vi "LoadConductusLTC-20c.vi"() -> ()   [LabVIEW 2020]
uses:
  <vilib>/Utility/file.llb/Read From Spreadsheet File (DBL).vi
panel:
  in  "Case Constant\n(See Context Help)":bool=TRUE
  out "ManyCal?":string="Too Many Calibration Entries"
  out "Sensor":string=":cernox 1030 X04981.cal2"
  out "Loading:":i32
  in  "More...":bool=TRUE
  out "CalArray":string[](array[string])=["325.000,2.02480,", "320.000,2.02830,", "310.000,2.03560,", "300.000,2.04330,", "290.000,2.05150,", "280.000,2.05960,", "270.000,2.06840,", "260.000,2.07700,", "250.000,2.08660,", "240.000,2.09600,", "230.000,2.10620,", "220.000,2.11640,", "210.000,2.12740,", "200.000,2.13890,", "190.000,2.15060,", "180.000,2.16290,", "170.000,2.17600,", "160.000,2.18960,", "150.000,2.20390,", "140.000,2.21930,", "130.000,2.23510,", "120.000,2.25180,", "110.000,2.26960,", "100.000,2.28870,", "90.000,2.30910,", "80.000,2.33160,", "77.350,2.33790,", "75.000,2.34350,", "70.000,2.35620,", "60.000,2.38390,", "56.000,2.39580,", "54.000,2.40200,", "50.000,2.41500,", "46.000,2.42910,", "44.000,2.43630,", "40.000,2.45170,", "38.000,2.45980,", "36.000,2.46820,", "34.000,2.47700,", "32.000,2.48650,", "30.000,2.49610,", "28.000,2.50610,", "26.000,2.51680,", "24.000,2.52810,", "22.000,2.54030,", "20.000,2.55340,", "19.000,2.56040,", "18.000,2.56750,", "17.000,2.57510,", "16.000,2.58310,", "15.000,2.59170,", "14.000,2.60120,", "13.000,2.61050,", "12.000,2.62100,", "11.000,2.63250,", "10.000,2.64480,", "9.500,2.65150,", "9.000,2.65880,", "8.500,2.66660,", "8.000,2.67440,", "7.500,2.68330,", "7.000,2.69270,", "6.500,2.70230,", "6.000,2.71370,", "5.800,2.71840,", "5.400,2.72870,", "5.000,2.73950,", "4.600,2.75160,", "4.200,2.76480,", "4.000,2.77230,", "3.900,2.77610,", "3.800,2.78000,", "3.700,2.78390,", "3.600,2.78810,", "3.500,2.79240,", "3.400,2.79700,", "3.300,2.80160,", "3.200,2.80650,", "3.100,2.81150,", "3.000,2.81660,", "2.900,2.82200,", "2.800,2.82780,", "2.700,2.83370,", "2.600,2.84000,", "2.500,2.84660,", "2.400,2.85350,", "2.300,2.86120,", "2.200,2.86870,", "2.100,2.87700,", "2.000,2.88560,", "1.900,2.89500,", "1.800,2.90520,", "1.700,2.91630,", "1.600,2.92920,", "1.500,2.94380,", "1.400,2.96020,", "1.300,2.97870,"]
  out "CharMatch":string="SCALT4,2,0,OptCernoxX02158,-1.0,"
  out "TempData":sgl[](array[numeric])=[325.0, 320.0, 310.0, 300.0, 290.0, 280.0, 270.0, 260.0, 250.0, 240.0, 230.0, 220.0, 210.0, 200.0, 190.0, 180.0, 170.0, 160.0, 150.0, 140.0, 130.0, 120.0, 110.0, 100.0, 90.0, 80.0, 77.35, 75.0, 70.0, 60.0, 56.0, 54.0, 50.0, 46.0, 44.0, 40.0, 38.0, 36.0, 34.0, 32.0, 30.0, 28.0, 26.0, 24.0, 22.0, 20.0, 19.0, 18.0, 17.0, 16.0, 15.0, 14.0, 13.0, 12.0, 11.0, 10.0, 9.5, 9.0, 8.5, 8.0, 7.5, 7.0, 6.5, 6.0, 5.8, 5.4, 5.0, 4.6, 4.2, 4.0, 3.9, 3.8, 3.7, 3.6, 3.5, 3.4, 3.3, 3.2, 3.1, 3.0, 2.9, 2.8, 2.7, 2.6, 2.5, 2.4, 2.3, 2.2, 2.1, 2.0, 1.9, 1.8, 1.7, 1.6, 1.5, 1.4, 1.3] format="%.2f"
  out "LogOhms":sgl[](array[numeric])=[2.0248, 2.0283, 2.0356, 2.0433, 2.0515, 2.0596, 2.0684, 2.077, 2.0866, 2.096, 2.1062, 2.1164, 2.1274, 2.1389, 2.1506, 2.1629, 2.176, 2.1896, 2.2039, 2.2193, 2.2351, 2.2518, 2.2696, 2.2887, 2.3091, 2.3316, 2.3379, 2.3435, 2.3562, 2.3839, 2.3958, 2.402, 2.415, 2.4291, 2.4363, 2.4517, 2.4598, 2.4682, 2.477, 2.4865, 2.4961, 2.5061, 2.5168, 2.5281, 2.5403, 2.5534, 2.5604, 2.5675, 2.5751, 2.5831, 2.5917, 2.6012, 2.6105, 2.621, 2.6325, 2.6448, 2.6515, 2.6588, 2.6666, 2.6744, 2.6833, 2.6927, 2.7023, 2.7137, 2.7184, 2.7287, 2.7395, 2.7516, 2.7648, 2.7723, 2.7761, 2.78, 2.7839, 2.7881, 2.7924, 2.797, 2.8016, 2.8065, 2.8115, 2.8166, 2.822, 2.8278, 2.8337, 2.84, 2.8466, 2.8535, 2.8612, 2.8687, 2.877, 2.8856, 2.895, 2.9052, 2.9163, 2.9292, 2.9438, 2.9602, 2.9787] format="%.2f"
  in  "Sensor BasePath":path=path "/Opticsmac/Thermometer Calibrations/ Optics"
  out "Sensor Path":path=path "/Opticsmac/Thermometer Calibrations/ Optics"
  in  "Load Curve":bool
  in  "Sensor Selection":u16(ring) items=["MultiSample30T", "MultiSample20T/Single Sample30T (head..)", "TransmissionProbe 30T", "Double Sample 30T", "SingleSample 30T", "Voigt-6SampleProbe 20T", "Nurmikko30T Top-emission", "Wim MOKE Probe"]
  in  "Sensor Array":T1(array[cluster])=[{"Sensor Path"=path "cernox 1030 X04981.cal2", "Sensor Info"="MultiSample30T"}, {"Sensor Path"=path "NML Opt Cernox X01971.cal", "Sensor Info"="MultiSample20T/Single Sample30T (head..)"}, {"Sensor Path"=path "cernox 1030 (x02158).rev", "Sensor Info"="TransmissionProbe 30T"}, {"Sensor Path"=path "NML-Opt Cernox X02363.cal2", "Sensor Info"="Double Sample 30T"}, {"Sensor Path"=path "", "Sensor Info"="SingleSample 30T"}, {"Sensor Path"=path "", "Sensor Info"="Voigt-6SampleProbe 20T"}, {"Sensor Path"=path "NML-Opt Cernox X04975.cal", "Sensor Info"="Nurmikko30T Top-emission"}, {"Sensor Path"=path "cernox 1010(x01974).rev", "Sensor Info"="Wim MOKE Probe"}]
  in  "LTC-20 BPIB":refnum<visa-resource-name>
  # "Tested successfully on S/N 0195"
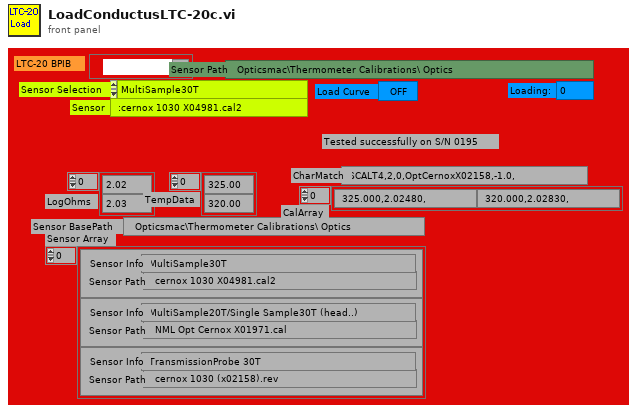
[diagram p1: front panel]
types:
  T1 = cluster{"Sensor Path":path, "Sensor Info":string}[]
  T2 = cluster{"Sensor Path":path, "Sensor Info":string}
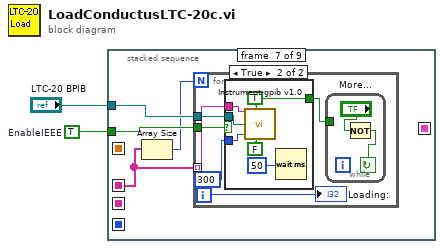
[diagram p0: block diagram]
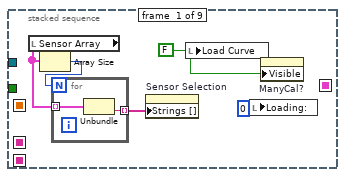
[diagram p2: hidden frame]
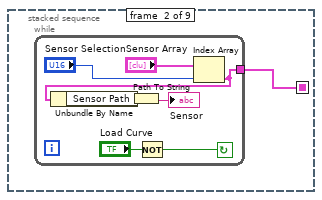
[diagram p3: hidden frame]
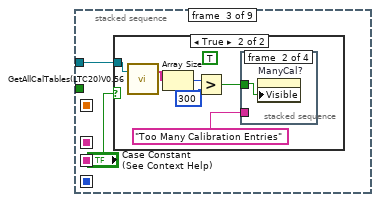
[diagram p4: hidden frame]
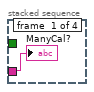
[diagram p6: hidden frame]
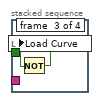
[diagram p7: hidden frame]
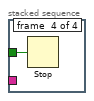
[diagram p8: hidden frame]
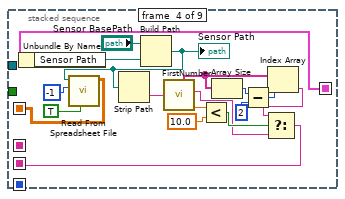
[diagram p9: hidden frame]
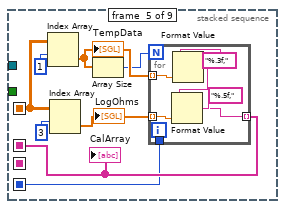
[diagram p10: hidden frame]
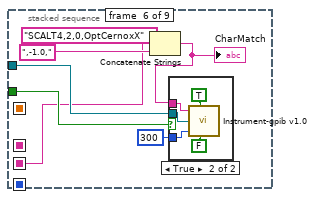
[diagram p11: hidden frame]
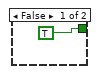
[diagram p13: hidden frame]
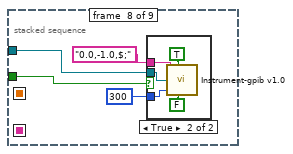
[diagram p14: hidden frame]
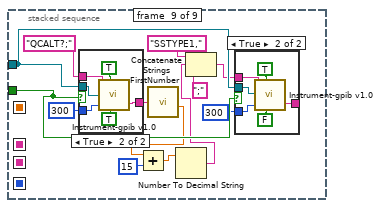
[diagram p16: hidden frame]
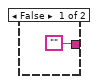
[diagram p17: hidden frame]
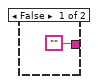
[diagram p18: hidden frame]
diagram:
  w2 = TRUE  # EnableIEEE
  n1 = stacked-sequence {
    seq-local: [_ w10 _ _ _ _ _ _ _] -> [_ _ _ w48 _ _ _ _ _]
    seq-local: [_ _ _ w45 _ _ _ _ _] -> [_ _ _ _ w54 _ _ _ _]
    seq-local: [_ _ _ _ w50 _ _ _ _] -> [_ _ _ _ _ _ w77 _ _]
    seq-local: [_ _ _ w31 _ _ _ _ _] -> [_ _ _ _ _ w65 _ _ _]
    seq-local: [_ _ _ _ w49 _ _ _ _] -> [_ _ _ _ _ _ _ _ _]
    tunnel: w2 -> [_ _ _ _ _ w68 w79 w97 w113]
    tunnel: "LTC-20 BPIB" -> [_ _ w19 _ _ w70 w78 w96 w114]
    frame #0 {
      w4 = FALSE
      n2 = local read "Sensor Array"() -> (w7:T1)
      n3 = Array Size(array=w7) -> (size(s)=w6:i32)
      n4 = for {
        N: w6 -> [_]
        tunnel: w7 -> [w9] mode=indexing
        tunnel: [w8] -> w5 mode=indexing
        n5 = Unbundle(w9) -> ("Sensor Info"=w8:string)  [unwired: 1 out]
      }
      n6 = property on="Sensor Selection" class="Ring (strict)"("Strings []"=w5) -> ()  [unwired: 2 in, 2 out]
      n7 = local write "Load Curve"(w4) -> ()
      n8 = local write "Loading:"(0) -> ()
      n9 = property on="ManyCal?" class="Str"("Visible"=w4) -> ()  [unwired: 2 in, 2 out]
    }
    frame #1 {
      n10 = while {
        tunnel: [w13] -> w10
        stop <- w16 continue-if-true
        n11 = Not(x="Load Curve") -> (.not. x?=w16:bool)
        n12 = Index Array(array="Sensor Array", index="Sensor Selection") -> (element=w13:T2)
        n13 = Unbundle By Name(w13) -> ("Sensor Path"=w12:path)
        n14 = Path To String(path=w12) -> (string=→"Sensor":string)
      }
    }
    frame #2 {
      n15 = case shown="True" "Case Constant\n(See Context Help)" {
        tunnel: w19 -> [_ w24]
        frame False {
        }
        frame True {
          (unwired) TRUE
          n16 = call "GetAllCalTables(LTC20)V0.56.vi"("LTC-20 IEEE"=w24) -> ("CalTables"=w25:string[])  [unwired: 1 in, 1 out]
          n17 = Array Size(array=w25) -> (size(s)=w21:i32)
          n18 = Greater?(x=w21, y=300) -> (0:w20:bool)
          n19 = stacked-sequence {
            tunnel: w20 -> [_ w27 w29 w30]
            tunnel: "Too Many Calibration Entries" -> [w26 _ _ _]
            frame #0 {
              "ManyCal?" <- w26
            }
            frame #1 {
              n20 = property on="ManyCal?" class="Str"("Visible"=w27) -> ()  [unwired: 2 in, 2 out]
            }
            frame #2 {
              n21 = Not(x=w29) -> (.not. x?=w28:bool)
              n22 = local write "Load Curve"(w28) -> ()
            }
            frame #3 {
              n23 = Stop(stop? (T)=w30) -> ()
            }
          }
        }
      }
    }
    frame #3 {
      n24 = Unbundle By Name(w48) -> ("Sensor Path"=w46:path)
      n25 = Build Path(base path="Sensor BasePath", name or relative path=w46) -> (appended path=w42:path)
      "Sensor Path" <- w42
      n26 = call-poly <vilib>:"Read From Spreadsheet File.vi"("transpose (no:F)"=TRUE, "number of rows (all:-1)"=-1, "file path (dialog if empty)"=w42) -> ("all rows"=w45:dbl[][])  [unwired: 4 in, 4 out]
      n27 = Strip Path(path=w42) -> (name=w41:string)  [unwired: 1 out]
      n28 = call "FirstNumber.vi"("Input String"=w41) -> ("Number Stings"=w38:string[], 4:"LastNumber"=w32:string, 6:"LastNumber"=w40:ext)  [unwired: 3 out]
      n29 = Less?(x=w40, y=10.0) -> (x < y?=w34:bool)
      n30 = Array Size(array=w38) -> (size(s)=w36:i32)
      n31 = Subtract(x=w36, y=2) -> (x-y=w37:i32)
      n32 = Index Array(array=w38, index=w37) -> (element=w33:string)
      n33 = Select(t=w33, s=w34, f=w32) -> (s? t:f=w31:string)
    }
    frame #4 {
      n34 = Index Array(array=w54, index (row)=1) -> (element=w53:dbl[])  [unwired: 1 in]
      "TempData" <- w53
      n35 = Index Array(array=w54, index (row)=3) -> (element=w52:dbl[])  [unwired: 1 in]
      "LogOhms" <- w52
      n36 = Array Size(array=w53) -> (size(s)=w51:i32)
      n37 = for {
        N: w51 -> [_]
        tunnel: w53 -> [w58] mode=indexing
        tunnel: w52 -> [w63] mode=indexing
        tunnel: [w60] -> w50 mode=indexing
        tunnel: [w57] -> w49
        i -> [w57]
        n38 = Format Value(format string="%.3f,", value (0)=w58) -> (output string=w59:string)  [unwired: 1 in]
        n39 = Format Value(string ("")=w59, format string="%.5f,", value (0)=w63) -> (output string=w60:string)
      }
      "CalArray" <- w50
    }
    frame #5 {
      n40 = Concatenate Strings("SCALT4,2,0,OptCernoxX", w65, ",-1.0,") -> (w64:string)
      "CharMatch" <- w64
      n41 = case shown="True" w68 {
        tunnel: 300 -> [_ w74]
        tunnel: w70 -> [_ w72]
        tunnel: w64 -> [_ w71]
        frame False {
        }
        frame True {
          n42 = call "Instrument-gpib v1.0.VI"("Characters to Write"=w71, "Write?"=TRUE, "GPIB Address"=w72, "Timeout (msec)"=w74, "Read?"=FALSE) -> ()  [unwired: 2 out]
        }
      }
    }
    frame #6 {
      n43 = Array Size(array=w77) -> (size(s)=w76:i32)
      n44 = for {
        N: w76 -> [_]
        tunnel: w78 -> [w85]
        tunnel: w79 -> [w83]
        tunnel: w77 -> [w82] mode=indexing
        i -> [w80]
        n45 = case shown="True" w83 {
          tunnel: 300 -> [_ w93]
          tunnel: w85 -> [_ w90]
          tunnel: w82 -> [_ w89]
          tunnel: [TRUE w92] -> w81
          frame False {
          }
          frame True {
            w92 = TRUE
            n46 = call "Instrument-gpib v1.0.VI"("Characters to Write"=w89, "Write?"=w92, "GPIB Address"=w90, "Timeout (msec)"=w93, "Read?"=FALSE) -> ()  [unwired: 2 out]
            n47 = Wait (ms)(milliseconds to wait=u32 50) -> ()  [unwired: 1 out]
          }
        }
        n48 = while {
          tunnel: w81 -> [_]
          stop <- w87 continue-if-true
          n49 = Not(x="More...") -> (.not. x?=w87:bool)
        }
        "Loading:" <- w80
      }
    }
    frame #7 {
      n50 = case shown="True" w97 {
        tunnel: 300 -> [_ w102]
        tunnel: w96 -> [_ w99]
        tunnel: "0.0,-1.0,$;" -> [_ w100]
        frame False {
        }
        frame True {
          n51 = call "Instrument-gpib v1.0.VI"("Characters to Write"=w100, "Write?"=TRUE, "GPIB Address"=w99, "Timeout (msec)"=w102, "Read?"=FALSE) -> ()  [unwired: 2 out]
        }
      }
    }
    frame #8 {
      n52 = case shown="True" w113 {
        tunnel: 300 -> [_ w129]
        tunnel: w114 -> [_ w126]
        tunnel: "QCALT?;" -> [_ w125]
        tunnel: ["" w127] -> w111
        frame False {
        }
        frame True {
          n53 = call "Instrument-gpib v1.0.VI"("Characters to Write"=w125, "Write?"=TRUE, "GPIB Address"=w126, "Timeout (msec)"=w129, "Read?"=TRUE) -> ("Characters Read"=w127:string)  [unwired: 1 out]
        }
      }
      n54 = call "FirstNumber.vi"("Input String"=w111) -> ("FirstNumber"=w106:ext)  [unwired: 5 out]
      n55 = Add(x=w106, y=15) -> (x+y=w105:ext)
      n56 = Number To Decimal String(number=w105) -> (decimal integer string=w104:string)  [unwired: 1 in]
      n57 = Concatenate Strings("SSTYPE1,", w104, ";") -> (w109:string)
      n58 = case shown="True" w113 {
        tunnel: 300 -> [_ w122]
        tunnel: w114 -> [_ w118]
        tunnel: w109 -> [_ w119]
        tunnel: ["" w120] -> _
        frame False {
        }
        frame True {
          n59 = call "Instrument-gpib v1.0.VI"("Characters to Write"=w119, "Write?"=TRUE, "GPIB Address"=w118, "Timeout (msec)"=w122, "Read?"=FALSE) -> ("Characters Read"=w120:string)  [unwired: 1 out]
        }
      }
    }
  }
